vi "LSS Parse.vi"(8 "Error in":errorcluster, 11 "Style Sheet":string) -> (0 "Error out":errorcluster, 3 "LSS Styles":T1[](array[typedef]))   [LabVIEW 2019, in "LSS.lvlib"]
doc: "This VI takes the input Style Sheet and outputs a cluster of information containing the information from the style sheet parsed into a useable format. If the style sheet does not follow the standard conventions this will return an error indicating what is wrong with the style sheet.\n\nInputs:\n<b>Style Sheet Text</b> - Text either from a string constant or file directly input.\n<b>Error In</b> - Error in terminal\n\nOutputs:\n<b>Style Sheet</b> - Array of clusters containing the information from the style sheet.\n<b>Error Out</b> - Error out terminal"
uses:
  LSS.lvlib
  Controls/Style.ctl
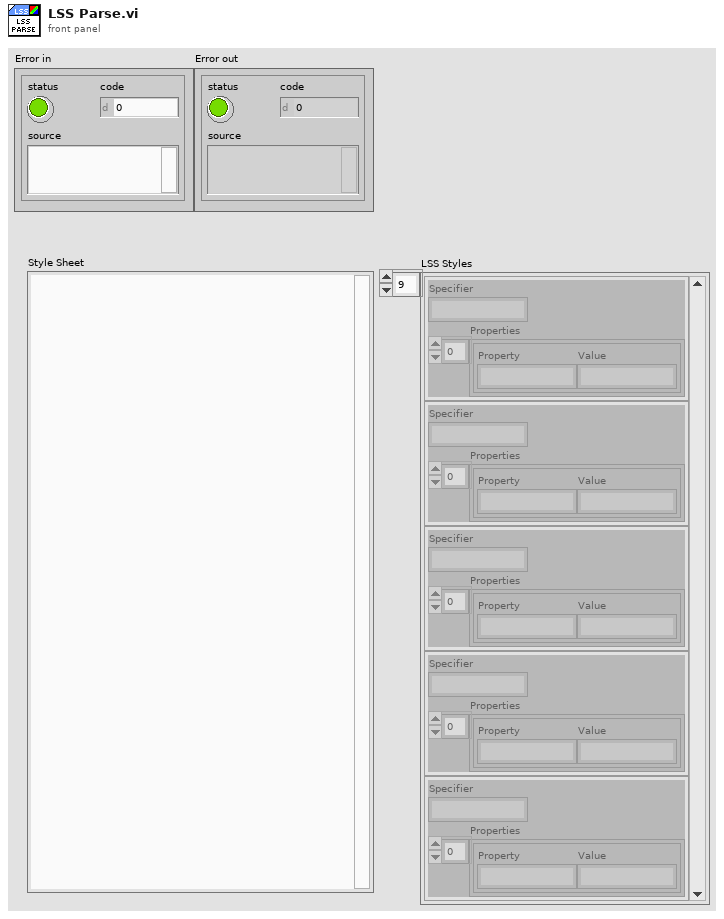
[diagram p1: front panel]
types:
  T1 = typedef "LSS.lvlib/Style.ctl" = cluster{"Specifier":string, "Properties":cluster{"Property":string, "Value":string}[]}
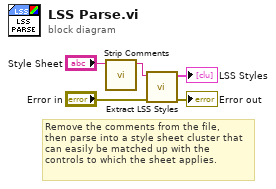
[diagram p0: block diagram]
diagram:
  # "Remove the comments from the file,\nthen parse into a style sheet cluster that\ncan easily be matched up with the\ncontrols to which the sheet applies."
  n1 = call "Strip Comments.vi"("File In"="Style Sheet") -> ("File Without Comments"=w5:string)  [unwired: 10 in]
  n2 = call "Extract LSS Styles.vi"("Error in"="Error in", "File Without Comments"=w5) -> ("Error out"=→"Error out":errorcluster, "LSS Styles"=→"LSS Styles":T1[])  [unwired: 8 in]
